vi "1_1.vi"() -> ()   [LabVIEW 2019]
doc: "Use this template to simulate the generation and display of data.\nNote: LabVIEW enables automatic error handling by default for VIs you create from this template."
uses:
  Instance           1 27Saved   GenerateDisplay.vit .vi
panel:
  in  "Amplitude":sgl(knob) scale=0.0..5.0
  out "Waveform Graph":dynamicdata(graph)
  in  "stop":bool
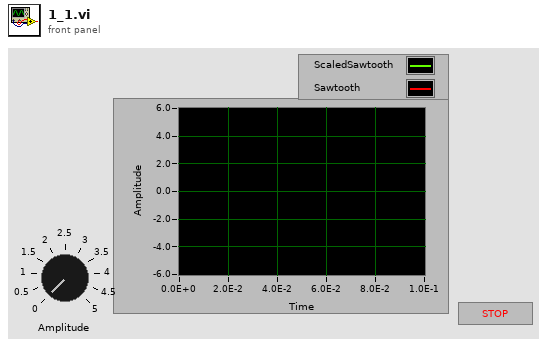
[diagram p1: front panel]
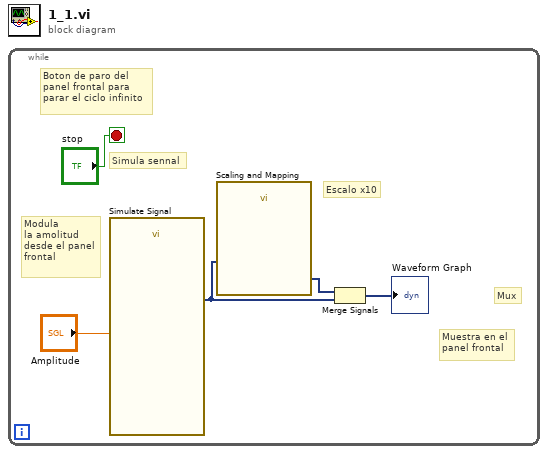
[diagram p0: block diagram]
diagram:
  n1 = while {
    stop <- "stop" stop-if-true
    # "Modula\nla amolitud\ndesde el panel\nfrontal"
    # "Escalo x10"
    # "Mux"
    # "Boton de paro del\npanel frontal para\nparar el ciclo infinito"
    # "Muestra en el\npanel frontal"
    # "Simula sennal"
    n2 = call "Simulate Signal"("Amplitude"="Amplitude") -> ("Sawtooth"=w1:dynamicdata)  [unwired: 13 in, 1 out]
    n3 = call "Scaling and Mapping"("Signals"=w1) -> ("Scaled Signals"=w3:dynamicdata)  [unwired: 9 in, 1 out]
    n4 = Merge Signals(w3, w1) -> (→"Waveform Graph":dynamicdata)
  }
